vi "Auto Drive.vi"(9 "seconds":dbl, 10 "forward?":bool) -> ()   [LabVIEW 2019]
uses:
  Robot Global Data.vi
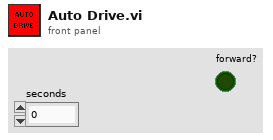
[diagram p1: front panel]
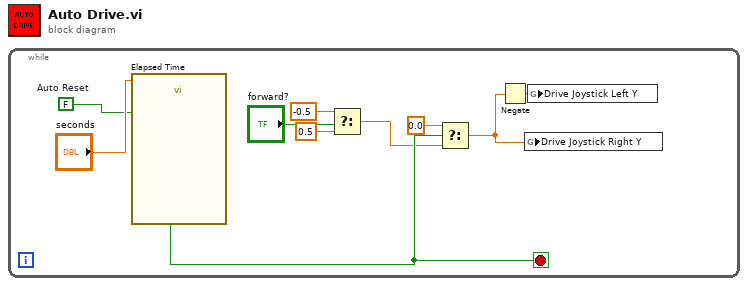
[diagram p0: block diagram]
diagram:
  n1 = while {
    stop <- w4 stop-if-true
    w5 = FALSE  # Auto Reset
    n2 = call "Elapsed Time"("Time Target (s)"="seconds", "Auto Reset"=w5) -> ("Time has Elapsed"=w4:bool)  [unwired: 10 in, 7 out]
    n3 = Select(t=-0.5, s="forward?", f=0.5) -> (s? t:f=w3:dbl)
    n4 = Select(t=0.0, s=w4, f=w3) -> (s? t:f=w1:dbl)
    n5 = Negate(x=w1) -> (-x=w10:dbl)
    n6 = global write "Robot Global Data.vi" "Drive Joystick Right Y"(w1) -> ()
    n7 = global write "Robot Global Data.vi" "Drive Joystick Left Y"(w10) -> ()
  }
